vi "create.messages.from.params.vi"(9 "Message.to.Create":refnum<class "MessageBase.lvclass">[](array[class]), 10 "Max.Frame.Size":u16=1500, 11 "Messages to Create":T1[](array[typedef])) -> (3 "Messages.Out":refnum<class "SequencedUnitHeader.lvclass">[](array[class]))   [LabVIEW 2020]
uses:
  pitch/SequencedUnitHeader/SequencedUnitHeader.lvclass
  pitch/MessageBase/MessageBase.lvclass
  pitch/ModifyOrder/ModifyOrderLong.lvclass
  pitch/oldMessageType.ctl
  Message.Spec.ctl
  pitch/SequencedUnitHeader/SequencedUnitHeader.Parameters.ctl
  pitch/Time/Time.Parameters.ctl
  pitch/Time/Time.lvclass
  pitch/AddOrder/AddOrderLong.Parameters.ctl
  pitch/AddOrder/AddOrderLong.lvclass
  pitch/ModifyOrder/ModifyOrderLong.Parameters.ctl
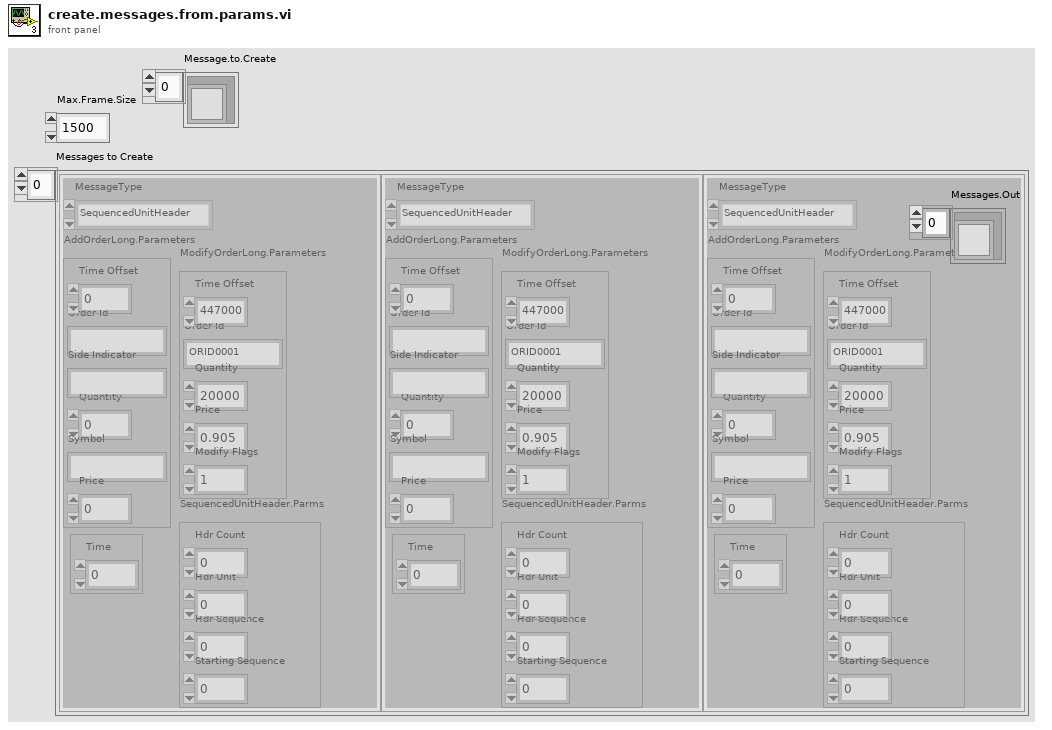
[diagram p1: front panel]
types:
  T1 = typedef "Message.Spec.ctl" = cluster{"MessageType":T2, "AddOrderLong.Parameters":T3, "Time.Parms":T4, "SequencedUnitHeader.Parms":T5, "ModifyOrderLong.Parameters":T6}
  T2 = typedef "oldMessageType.ctl" = enum16{"Time", "SequencedUnitHeader", "AddOrderLong", "AddOrderShort", "AddOrderExpanded", "ModifyOrderLong"}
  T3 = typedef "AddOrderLong.lvclass/AddOrderLong.Parameters.ctl" = cluster{"Time Offset":u32, "Order Id":string, "Quantity":u32, "Symbol":string, "Side Indicator":string, "Price":dbl}
  T4 = typedef "Time.lvclass/Time.Parameters.ctl" = cluster{"Time":u32}
  T5 = typedef "SequencedUnitHeader.lvclass/SequencedUnitHeader.Parameters.ctl" = cluster{"Hdr Count":u8, "Hdr Unit":u8, "Hdr Sequence":u32, "Starting Sequence":u32}
  T6 = typedef "ModifyOrderLong.lvclass/ModifyOrderLong.Parameters.ctl" = cluster{"Time Offset":u32, "Order Id":string, "Quantity":u32, "Price":dbl, "Modify Flags":u8}
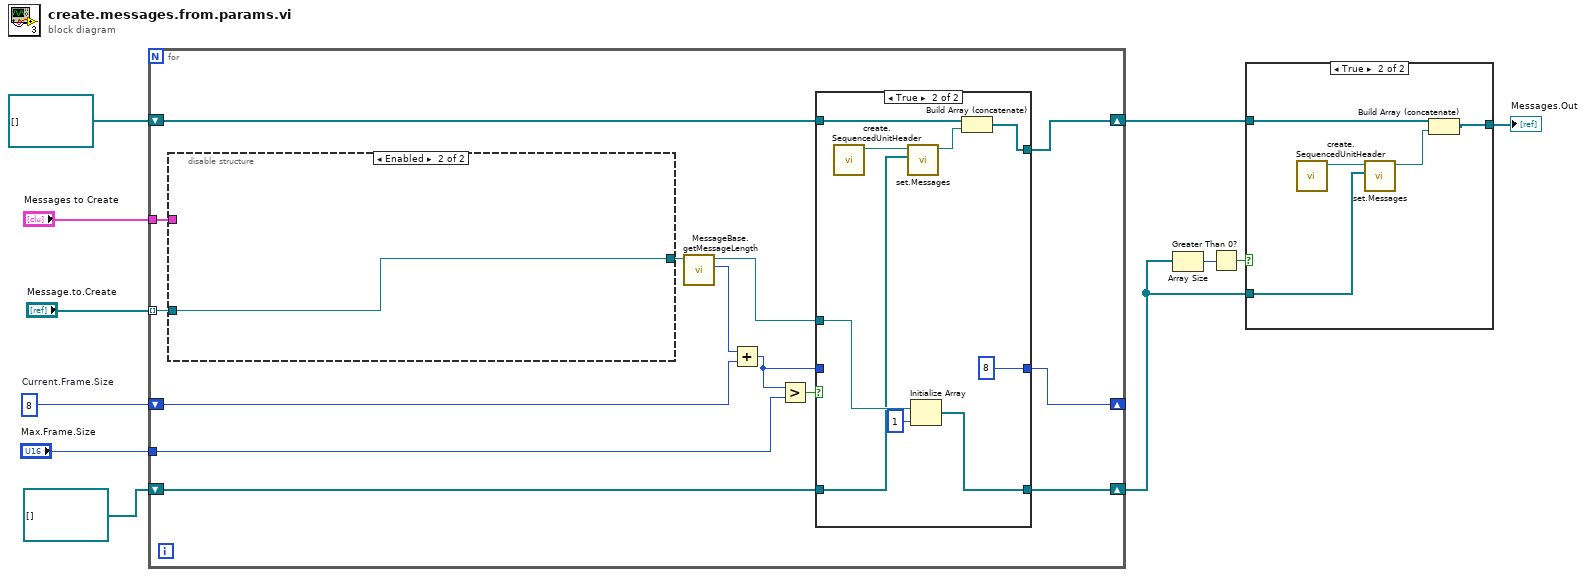
[diagram p0: block diagram]
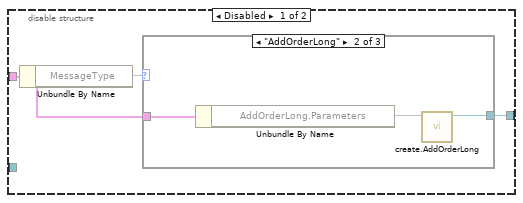
[diagram p3: hidden frame]
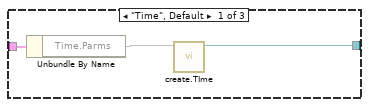
[diagram p4: hidden frame]
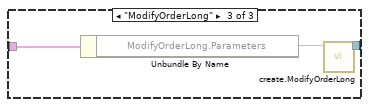
[diagram p5: hidden frame]
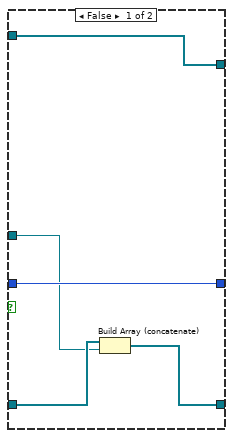
[diagram p6: hidden frame]
diagram:
  w10 = u16 8  # Current.Frame.Size
  n1 = for {
    tunnel: "Messages to Create" -> [w25]
    tunnel: "Max.Frame.Size" -> [w23]
    shift-right: [w21] -> _
    shift-left: w10 -> [w24]
    shift-right: [w18] -> w4
    shift-left: refnum<class "MessageBase.lvclass">[] [] -> [w19]
    shift-right: [w16] -> w3
    shift-left: refnum<class "SequencedUnitHeader.lvclass">[] [] -> [w17]
    tunnel: "Message.to.Create" -> [w12] mode=indexing
    n2 = disable-structure shown="Enabled" {
      disable-tunnel: w25 -> [w27 _]
      disable-tunnel: [w26 w38] -> w15
      disable-tunnel: w12 -> [_ w38]
      frame Disabled {
        n3 = Unbundle By Name(w27) -> ("MessageType"=w28)
        n4 = case shown="\"AddOrderLong\"" w28 {
          tunnel: w27 -> [w31 w34 w36]
          tunnel: [w29 w32 w37] -> w26
          frame "Time", Default {
            n5 = Unbundle By Name(w31) -> ("Time.Parms"=w30)
            n6 = call "create.TIme.vi"("Time.Parameters"=w30) -> ("MessageBase out"=w29:refnum<class "MessageBase.lvclass">)  [unwired: 8 in, 2 out]
          }
          frame "AddOrderLong" {
            n7 = Unbundle By Name(w34) -> ("AddOrderLong.Parameters"=w33)
            n8 = call "create.AddOrderLong.vi"("AddOrderLong.Parameters"=w33) -> ("MessageBase out"=w32:refnum<class "MessageBase.lvclass">)  [unwired: 9 in, 1 out]
          }
          frame "ModifyOrderLong" {
            n9 = Unbundle By Name(w36) -> ("ModifyOrderLong.Parameters"=w35)
            n10 = call "create.ModifyOrderLong.vi"("ModifyOrderLong.Parameters"=w35) -> ("MessageBase out"=w37:refnum<class "ModifyOrderLong.lvclass">)  [unwired: 8 in, 2 out]
          }
        }
      }
      frame Enabled {
      }
    }
    n11 = call-dynamic "MessageBase.getMessageLength.vi"("MessageBase in"=w15) -> ("Length"=w13:u8, "MessageBase out"=w14:refnum<class "MessageBase.lvclass">)  [unwired: 8 in, 1 out]
    n12 = Add(x=w13, y=w24) -> (x+y=w20:u16)
    n13 = Greater?(x=w20, y=w23) -> (0:w22:bool)
    n14 = case shown="True" w22 {
      tunnel: [w43 u16 8] -> w21
      tunnel: w20 -> [w43 _]
      tunnel: w19 -> [w42 w48]
      tunnel: w14 -> [w41 w51]
      tunnel: [w40 w50] -> w18
      tunnel: w17 -> [w39 w46]
      tunnel: [w39 w45] -> w16
      frame False {
        n15 = Build Array (concatenate)(w42, w41) -> (w40:refnum<class "MessageBase.lvclass">[])
      }
      frame True {
        n16 = call "create.SequencedUnitHeader.vi"() -> ("PitchMessage out"=w49:refnum<class "SequencedUnitHeader.lvclass">)  [unwired: 10 in, 1 out]
        n17 = call-dynamic "set.Messages.vi"("Messages.In"=w48, "SequencedUnitHeader in"=w49) -> ("SequencedUnitHeader out"=w47:refnum<class "SequencedUnitHeader.lvclass">)  [unwired: 8 in, 1 out]
        n18 = Initialize Array(w51, 1 ("dimension size")) -> (w50:refnum<class "MessageBase.lvclass">[])
        n19 = Build Array (concatenate)(w46, w47) -> (w45:refnum<class "SequencedUnitHeader.lvclass">[])
      }
    }
  }
  n20 = Array Size(array=w4) -> (size(s)=w6:i32)
  n21 = Greater Than 0?(x=w6) -> (x > 0?=w5:bool)
  n22 = case shown="True" w5 {
    tunnel: w4 -> [_ w57]
    tunnel: w3 -> [w53 w55]
    tunnel: [w53 w54] -> w2
    frame False {
    }
    frame True {
      n23 = call "create.SequencedUnitHeader.vi"() -> ("PitchMessage out"=w58:refnum<class "SequencedUnitHeader.lvclass">)  [unwired: 10 in, 1 out]
      n24 = call-dynamic "set.Messages.vi"("Messages.In"=w57, "SequencedUnitHeader in"=w58) -> ("SequencedUnitHeader out"=w56:refnum<class "SequencedUnitHeader.lvclass">)  [unwired: 8 in, 1 out]
      n25 = Build Array (concatenate)(w55, w56) -> (w54:refnum<class "SequencedUnitHeader.lvclass">[])
    }
  }
  "Messages.Out" <- w2
